vi "novoGoleiroRotacionar.vi"(9 "balls":T1[](array[typedef]), 10 "Robot in":T2, 11 "IA State":T7={"our_robots"=[], "enemy_robots"=[], "balls"=[], "geometry"={"field_length"=0, "field_width"=0, "goal_width"=0, "goal_depth"=0, "center_circle_radius"=0, "defense_width"=0, "defense_depth"=0, "free_kick_from_defense_dist"=0, "penalty_spot_from_field_line_dist"=0, "penalty_line_from_spot_dist"=0, "half_moon_depth"=0, "half_moon_width"=0}, "IA Judge"={"stage"="", "command"="", "our_goalie_id"=0.0, "enemy_goalie_id"=0.0, "command enum"=enum."Halt", "Time"=enum."Azul"}, "Received Timestamp"=timestamp(0 s since 1904-01-01), "Events"={"Touch"=FALSE, "id touch"=0.0, "Ball out of \nVision"=FALSE, "Ball inside \nGoalie area"=FALSE, "Robot not responding"=FALSE, "Robots responding status"=[1.0, 1.0, 1.0, 1.0, 1.0, 1.0], "Enemy Ball \nPossession"=FALSE, "Id ini Possession"=0.0, "Ball Possesion"=FALSE, "Id Possesion"=0.0, "Ball at\nour goal side"=FALSE, "Ball at\ntouchline"=FALSE, "Ball at\nenemy goal side"=FALSE}}) -> (3 "Cluster de saída":T2)   [LabVIEW 2018]
uses:
  Core/AI Input.ctl
  Core/AI Robot.ctl
  Intel/Functions Enum.ctl
  Intel/AttackerStates.ctl
  Path Planning/RRT/PathDests.ctl
  Path Planning/RRT/PathDest.ctl
  Core/AI Ball.ctl
  Core/Field Size.ctl
  Core/AI Judge.ctl
  Intel/Command Enum.ctl
  Util/Events/Events.ctl
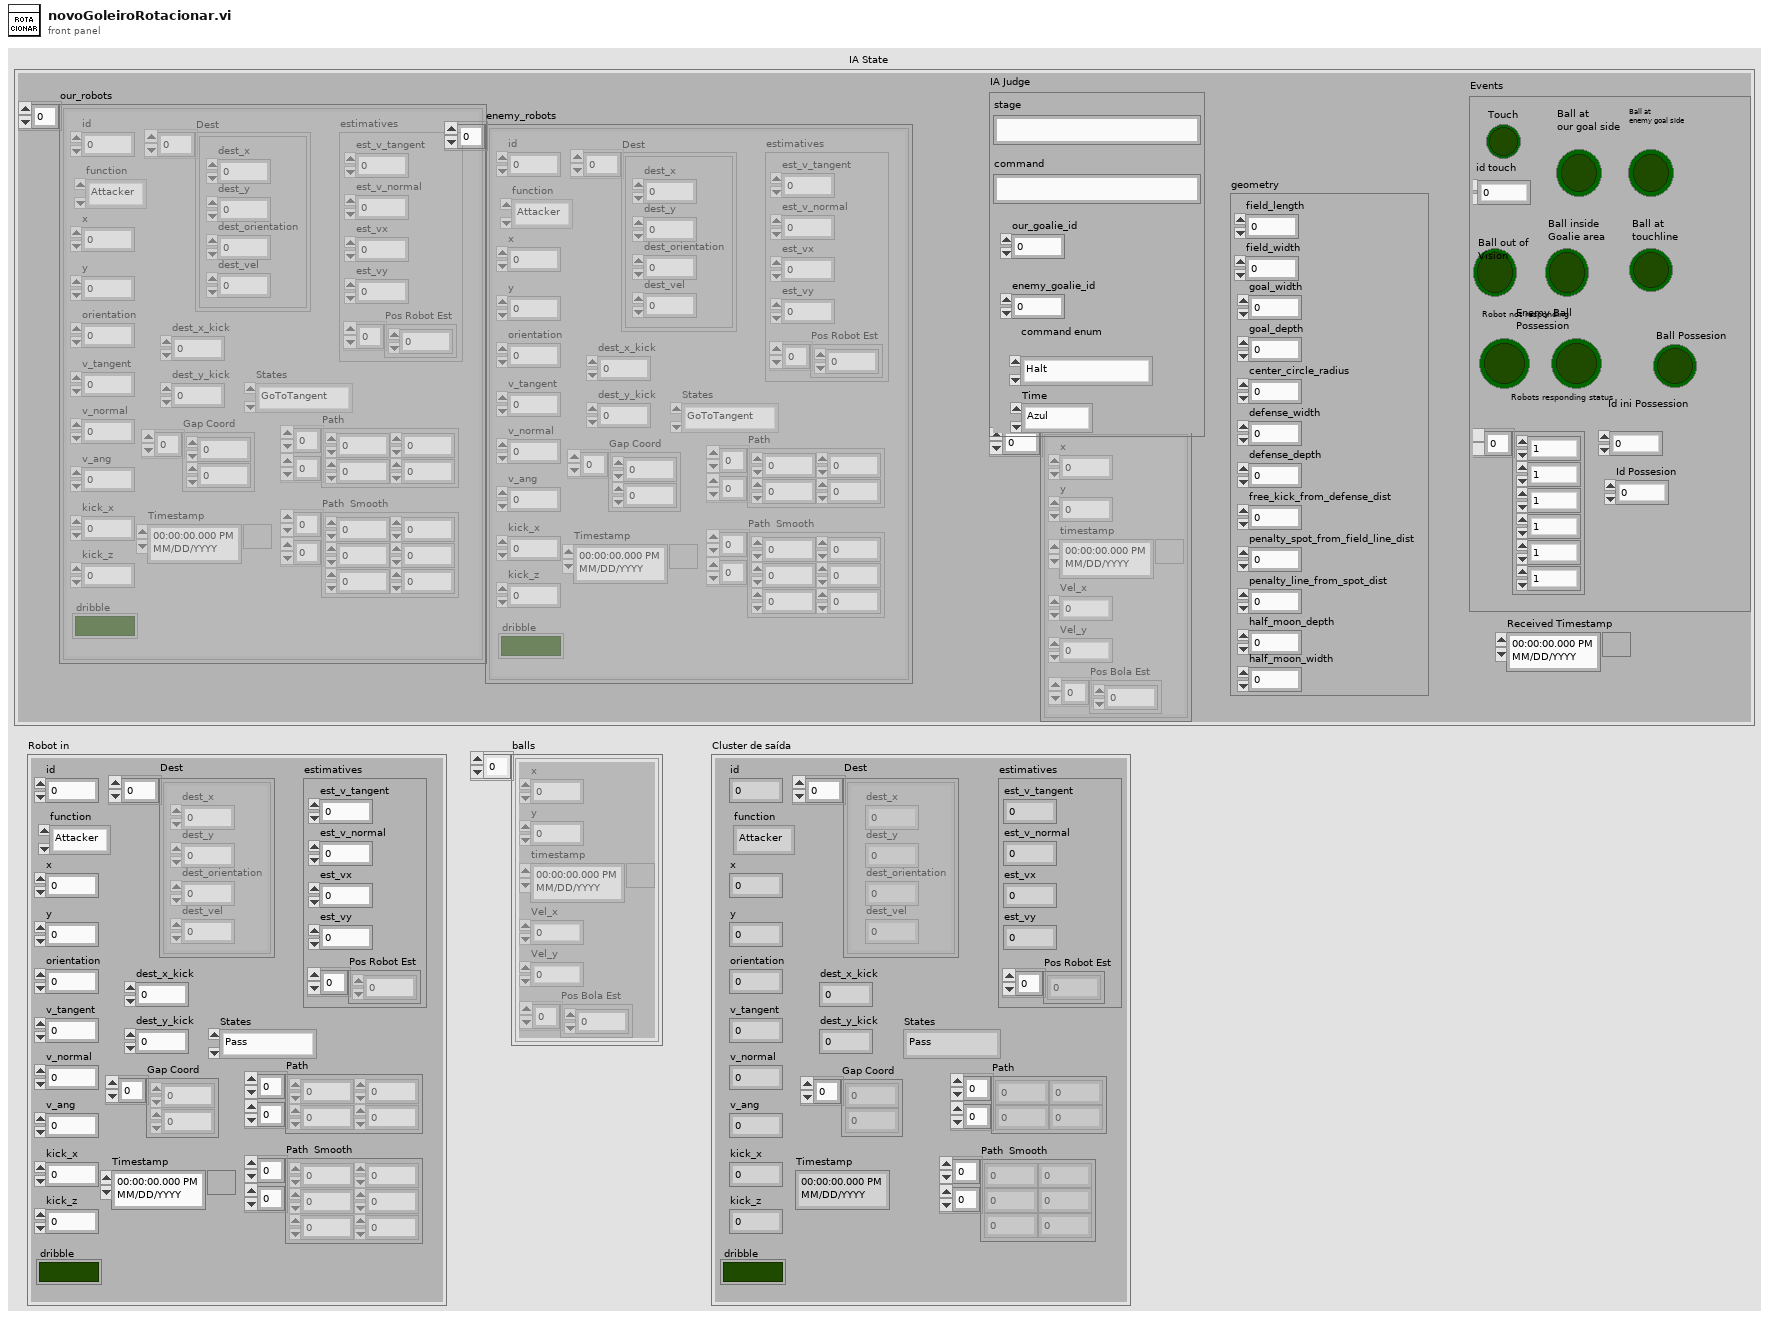
[diagram p1: front panel]
types:
  T1 = typedef "AI Ball.ctl" = cluster{"x":dbl, "y":dbl, "timestamp":timestamp, "Vel_x":dbl, "Vel_y":dbl, "Pos Bola Est":dbl[]}
  T2 = typedef "AI Robot.ctl" = cluster{"id":u32, "function":T3, "x":dbl, "y":dbl, "orientation":dbl, "v_tangent":dbl, "v_normal":dbl, "v_ang":dbl, "kick_x":dbl, "kick_z":dbl, "dribble":bool, "Timestamp":timestamp, "estimatives":cluster{"est_v_tangent":dbl, "est_v_normal":dbl, "est_vx":dbl, "est_vy":dbl, "Pos Robot Est":dbl[]}, "dest_x_kick":dbl, "dest_y_kick":dbl, "Gap Coord":dbl[], "States":T4, "Path ":dbl[][], "Path  Smooth":dbl[][], "Dest":T5}
  T3 = typedef "Functions Enum.ctl" = enum16{"Attacker", "Goalie", "Defender", "Striker", "Goto 0", "Dummy", "Kicker", "ZigZag"}
  T4 = typedef "AttackerStates.ctl" = enum16{"Pass", "GoToTangent", "BallGetting", "GoToKick", "Rotate anti-clockwise", "Rotate Clockwise", ""}
  T5 = typedef "PathDests.ctl" = T6[]
  T6 = typedef "PathDest.ctl" = cluster{"dest_x":dbl, "dest_y":dbl, "dest_orientation":dbl, "dest_vel":dbl}
  T7 = typedef "AI Input.ctl" = cluster{"our_robots":T2[], "enemy_robots":T2[], "balls":T1[], "geometry":T8, "IA Judge":T9, "Received Timestamp":timestamp, "Events":T11}
  T8 = typedef "Field Size.ctl" = cluster{"field_length":u32, "field_width":u32, "goal_width":u32, "goal_depth":u32, "center_circle_radius":u32, "defense_width":u32, "defense_depth":u32, "free_kick_from_defense_dist":u32, "penalty_spot_from_field_line_dist":u32, "penalty_line_from_spot_dist":u32, "half_moon_depth":u32, "half_moon_width":u32}
  T9 = typedef "AI Judge.ctl" = cluster{"stage":string, "command":string, "our_goalie_id":dbl, "enemy_goalie_id":dbl, "command enum":T10, "Time":enum16{"Azul", "Amarelo"}}
  T10 = typedef "Command Enum.ctl" = enum16{"Halt", "Stop", "Force Start", "PKA Normal Start", "Prepare Kickoff Ally", "PKE Normal Start", "Prepare Kickoff Enemy", "Prepare Penalty Ally", "PPA Normal Start", "Prepare Penalty Enemy", "PPE Normal Start", "Ball Placement Enemy Up", "Ball Placement Enemy Down", "Ball Placement Ally Up", "Ball Placement Ally Mid", "Ball Placement Ally Down", "Indirect Free Enemy", "Indirect Free Ally", "Timeout Enemy", "Timeout Ally", "Goal Enemy", "Goal Ally", "Normal Half Time", "Extra Time Break", "Extra Half Time", "None", "Post Game"}
  T11 = typedef "Events.ctl" = cluster{"Touch":bool, "id touch":dbl, "Ball out of \nVision":bool, "Ball inside \nGoalie area":bool, "Robot not responding":bool, "Robots responding status":dbl[], "Enemy Ball \nPossession":bool, "Id ini Possession":dbl, "Ball Possesion":bool, "Id Possesion":dbl, "Ball at\nour goal side":bool, "Ball at\ntouchline":bool, "Ball at\nenemy goal side":bool}
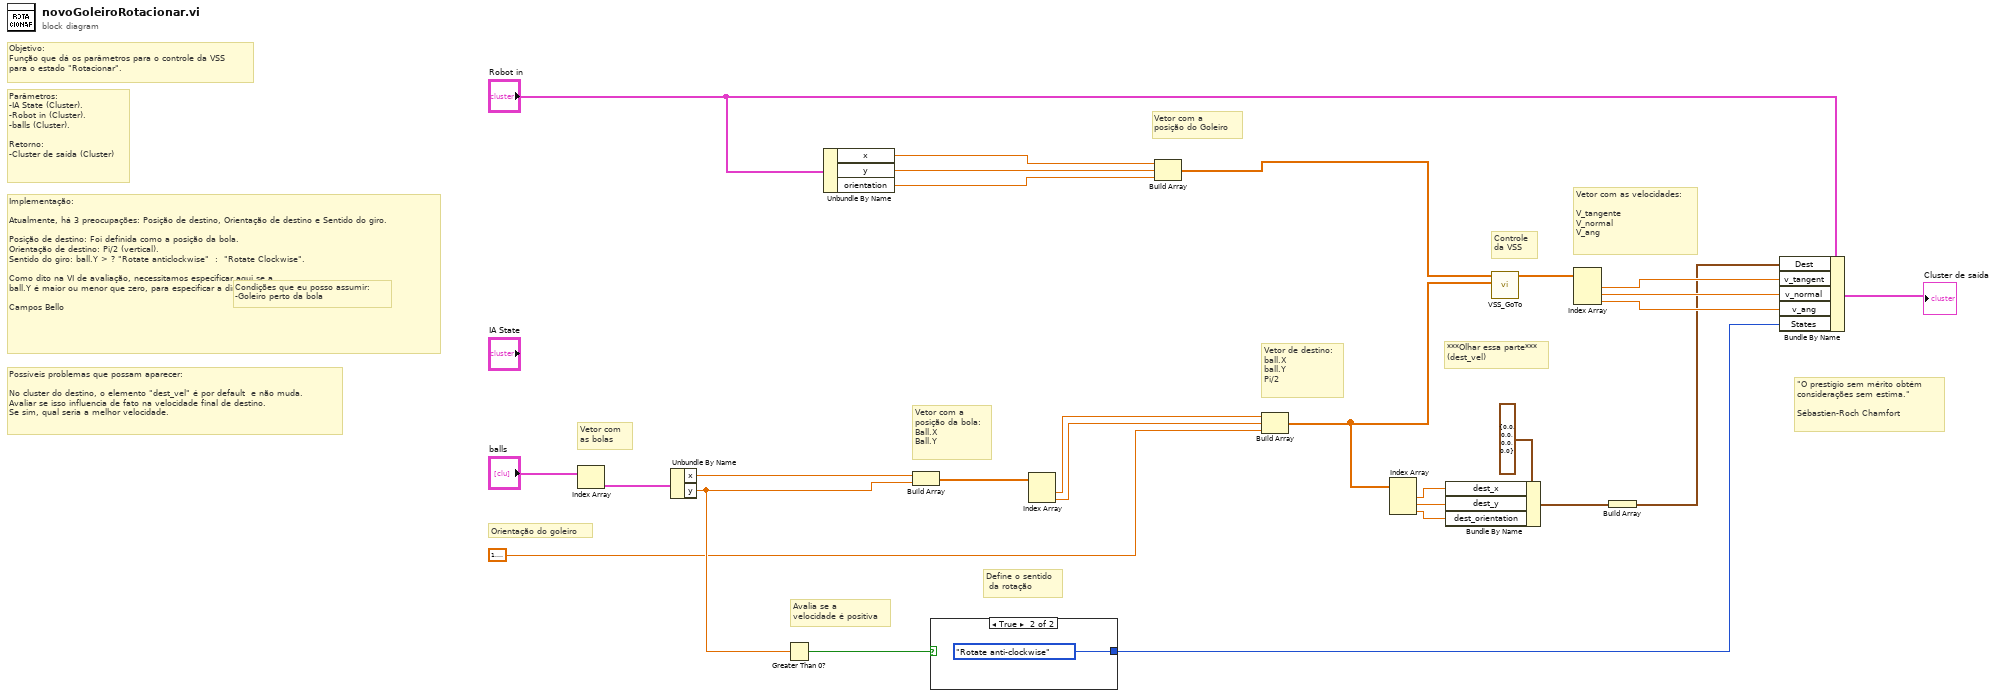
[diagram p0: block diagram]
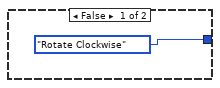
[diagram p2: hidden frame]
diagram:
  # "Orientação do goleiro"
  # "\"O prestígio sem mérito obtém \nconsiderações sem estima.\" \n\nSébastien-Roch Chamfort"
  # "Possíveis problemas que possam aparecer:\n\nNo cluster do destino, o elemento \"dest_vel\" é por default  e não muda. \nAvaliar se isso influencia de fato na velocidade final de destino.\nSe sim, qual seria a melhor velocidade."
  # "Implementação:\n\nAtualmente, há 3 preocupações: Posição de destino, Orientação de destino e Sentido do giro.\n\nPosição de destino: Foi definida como a posição da bola.\nOrientação de destino: Pi/2 (vertical).\nSentido do giro: ball.Y > ? \"Rotate anticlockwise\"  :  \"Rotate Clockwise\".\n\nComo dito na VI de avaliação, necessitamos especificar aqui se a \nball.Y é maior ou menor que zero, para especificar a direção do giro\n\nCampos Bello"
  # "Parâmetros:\n-IA State (Cluster).\n-Robot in (Cluster).\n-balls (Cluster).\n\nRetorno:\n-Cluster de saída (Cluster)"
  # "Objetivo:\nFunção que dá os parâmetros para o controle da VSS\npara o estado \"Rotacionar\"."
  # "Controle \nda VSS"
  # "***Olhar essa parte***\n(dest_vel)"
  # "Vetor com as velocidades:\n\nV_tangente\nV_normal\nV_ang"
  # "Vetor de destino:\nball.X\nball.Y\nPi/2"
  # "Vetor com a \nposição da bola:\nBall.X\nBall.Y"
  # "Define o sentido\n da rotação"
  # "Avalia se a \nvelocidade é positiva"
  # "Vetor com \nas bolas"
  # "Condições que eu posso assumir:\n-Goleiro perto da bola"
  # "Vetor com a \nposição do Goleiro"
  n1 = Index Array(array="balls") -> (element=w26:T1)  [unwired: 1 in]
  n2 = Unbundle By Name(w26) -> ("x"=w24:dbl, "y"=w23:dbl)
  n3 = Greater Than 0?(x=w23) -> (x > 0?=w25:bool)
  n4 = Unbundle By Name("Robot in") -> ("x"=w27:dbl, "y"=w2:dbl, "orientation"=w1:dbl)
  n5 = Build Array(w24, w23) -> (w22:dbl[])
  n6 = case shown="True" w25 {
    tunnel: [AttackerStates."Rotate Clockwise" ("States") AttackerStates."Rotate anti-clockwise" ("States")] -> w16
    frame False {
    }
    frame True {
    }
  }
  n7 = Index Array(array=w22) -> (element #1=w4:dbl, element #2=w3:dbl)  [unwired: 2 in]
  n8 = Build Array(w27, w2, w1) -> (w21:dbl[])
  n9 = Build Array(w4, w3, 1.5707963267948966) -> (w14:dbl[])
  n10 = Index Array(array=w14) -> (element #1=w13:dbl, element #2=w12:dbl, element #3=w11:dbl)  [unwired: 3 in]
  n11 = Bundle By Name(cluster=T6 {"dest_x"=0.0, "dest_y"=0.0, "dest_orientation"=0.0, "dest_vel"=0.0} ("element"), "dest_x"=w13, "dest_y"=w12, "dest_orientation"=w11) -> (w10:T6)
  n12 = call "VSS_GoTo.vi"("SetPoint"=w14, "Position"=w21) -> ("Output Vel"=w20:dbl[])  [unwired: 9 in]
  n13 = Index Array(array=w20) -> (element #1=w19:dbl, element #2=w18:dbl, element #3=w17:dbl)  [unwired: 3 in]
  n14 = Build Array(w10) -> (w9:T6[])
  n15 = Bundle By Name(cluster="Robot in", "Dest"=w9, "v_tangent"=w19, "v_normal"=w18, "v_ang"=w17, "States"=w16) -> (→"Cluster de saída":T2)
